vi "cast_ray.vi"(9 "Direction":dbl[](array[numeric]), 10 "Origin":dbl[](array[numeric]), 11 "Sphere":cluster{"Center":dbl[], "Radius":dbl}) -> (3 "Color":u32)   [LabVIEW 2015]
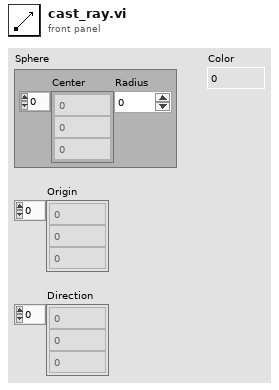
[diagram p1: front panel]
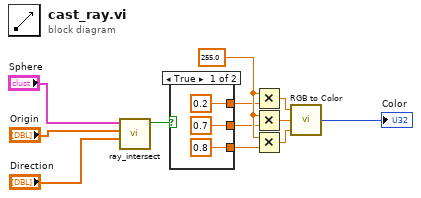
[diagram p0: block diagram]
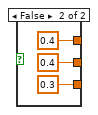
[diagram p2: hidden frame]
diagram:
  w4 = 255.0 ("x")
  n1 = call "ray_intersect.vi"("Direction"="Direction", "Origin"="Origin", "Sphere"="Sphere") -> ("RayIntersect"=w12:bool)  [unwired: 8 in]
  n2 = case shown="True" w12 {
    tunnel: [0.2 0.4] -> w3
    tunnel: [0.7 0.4] -> w2
    tunnel: [0.8 0.3] -> w1
    frame True {
    }
    frame False {
    }
  }
  n3 = Multiply(x=w4, y=w3) -> (x*y=w6:dbl)
  n4 = Multiply(x=w4, y=w2) -> (x*y=w7:dbl)
  n5 = Multiply(x=w4, y=w1) -> (x*y=w8:dbl)
  n6 = call <vilib>:"RGB to Color.vi"("B"=w8, "G"=w7, "R"=w6) -> ("Color"=→"Color":u32)
